vi "Simple AAP.vi"() -> ()   [LabVIEW 2013]
panel:
  out "Average Value":dbl
  out "Waveform Graph":dynamicdata(graph)
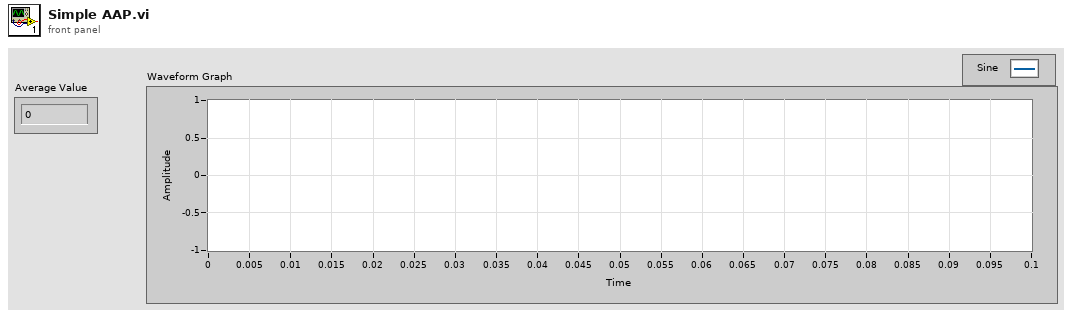
[diagram p1: front panel]
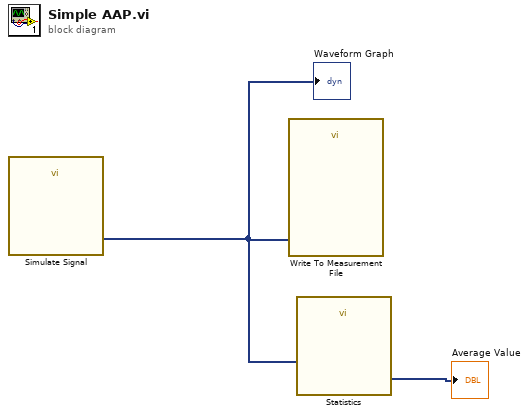
[diagram p0: block diagram]
diagram:
  n1 = call "Simulate Signal"() -> ("Sine"=w2:dynamicdata)  [unwired: 14 in, 1 out]
  "Waveform Graph" <- w2
  n2 = call "Write To Measurement File"("Signals"=w2) -> ()  [unwired: 16 in, 3 out]
  n3 = call "Statistics"("Signals"=w2) -> ("Arithmetic Mean"=→"Average Value":dynamicdata)  [unwired: 25 in, 1 out]
